vi "RandomNumberVI.vi"(8 "Lower Limit":dbl, 11 "Upper Limit":dbl) -> (0 "Random Number DBL":dbl, 1 "Random Number I8":i8, 2 "Random Number I16":i16, 3 "Random Number I32":i32)   [LabVIEW 2015]
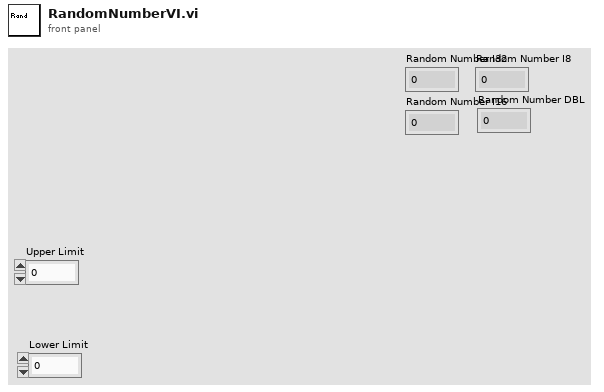
[diagram p1: front panel]
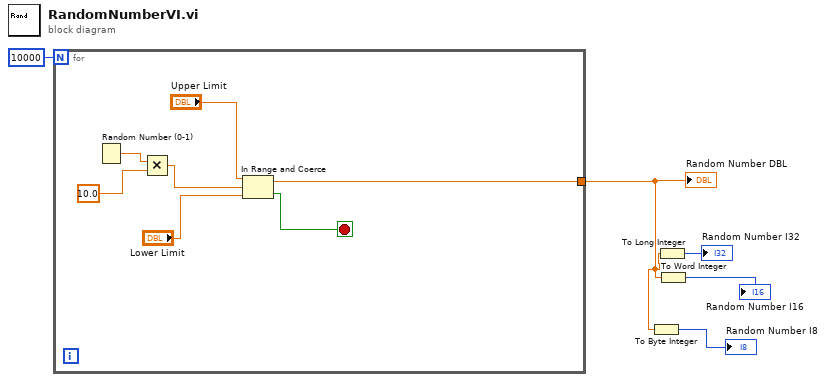
[diagram p0: block diagram]
diagram:
  n1 = for {
    N: 10000 -> [_]
    tunnel: [w6] -> w2
    stop <- w7 stop-if-true
    n2 = Random Number (0-1)() -> (number: 0 to 1=w10:dbl)
    n3 = Multiply(x=w10, y=10.0) -> (x*y=w8:dbl)
    n4 = In Range and Coerce(upper limit="Upper Limit", x=w8, lower limit="Lower Limit") -> (coerced(x)=w6:dbl, In Range?=w7:bool)
  }
  "Random Number DBL" <- w2
  n5 = To Byte Integer(number=w2) -> (8bit integer=→"Random Number I8":i8)
  n6 = To Long Integer(number=w2) -> (32bit integer=→"Random Number I32":i32)
  n7 = To Word Integer(number=w2) -> (16bit integer=→"Random Number I16":i16)
